vi "oneDtext2array(dbl).vi"(11 "String":string="\\voltsPerGram.txt") -> (3 "array":dbl[](array[numeric]))   [LabVIEW 2017]
uses:
  <vilib>/Utility/file.llb/Read Delimited Spreadsheet (DBL).vi
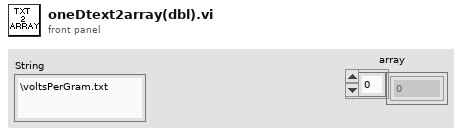
[diagram p1: front panel]
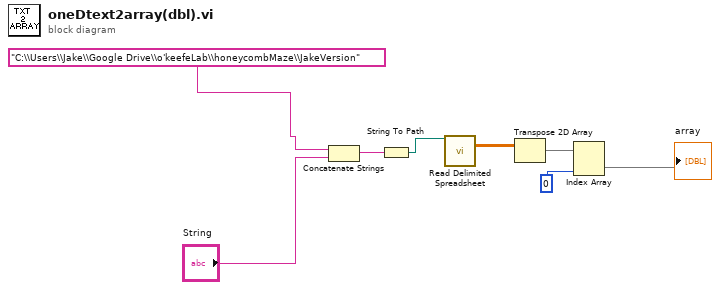
[diagram p0: block diagram]
diagram:
  n1 = Concatenate Strings("C:\\Users\\Jake\\Google Drive\\o'keefeLab\\honeycombMaze\\JakeVersion", "String") -> (w4:string)
  n2 = String To Path(string=w4) -> (path=w3:path)
  n3 = call-poly <vilib>:"Read Delimited Spreadsheet.vi"("file path (dialog if empty)"=w3) -> ("all rows"=w8:dbl[][])  [unwired: 9 in, 5 out]
  n4 = Transpose 2D Array(2D array=w8) -> (transposed array=w7:dbl[][])
  n5 = Index Array(array=w7, index (col)=0) -> (element=→"array":dbl[])  [unwired: 1 in]
